vi "FTW-ERR-UnknownParameter.vi"(7 "Unknown Parameter":string, 11 "error in":errorcluster) -> (15 "error out":errorcluster)   [LabVIEW 2013]
panel:
  # "Inputs"
  # "Outputs"
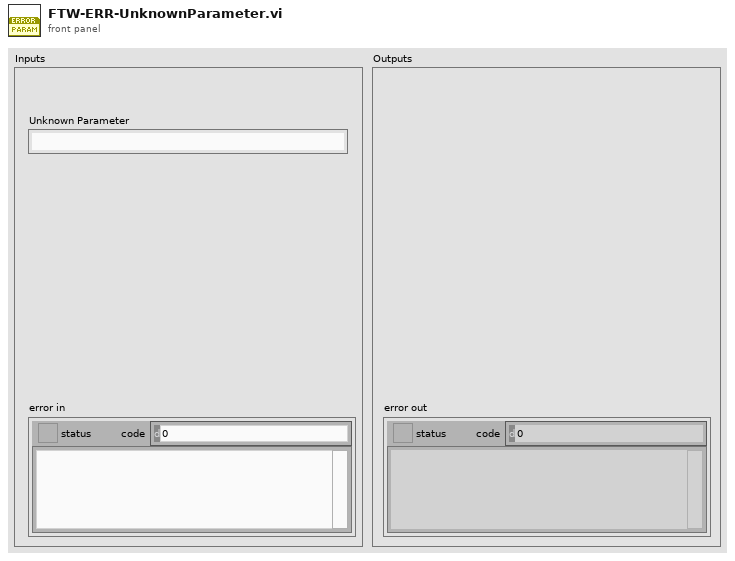
[diagram p1: front panel]
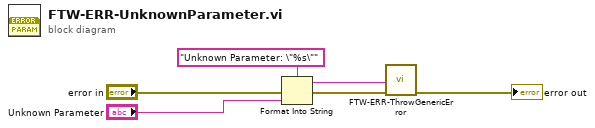
[diagram p0: block diagram]
diagram:
  n1 = Format Into String(format string="Unknown Parameter: \"%s\"", error in="error in", "Unknown Parameter") -> (resulting string=w2:string, error out=w3:errorcluster)  [unwired: 1 in]
  n2 = call "FTW-ERR-ThrowGenericError.vi"("Error Message"=w2, "error in"=w3) -> ("error out"=→"error out":errorcluster)  [unwired: 13 in]
